vi "OpticsSS.vi"   [LabVIEW 2019]
uses:
  OpticsSS.ctl
types:
  T1 = typedef "OpticsSS.ctl" = enum16{"_Quit_", "Init", "Ready", "HTL", "CCD_shot", "QueueData", "Error Handler", "HTL Error", "CCD Error", "CCDSetup", "Calibration", "BG_Setup", "HTL Paras Setup"}
  T2 = enum16{"CCDSetup", "Calibration", "BGShot", "SequenceShot", "SingleShot", "default"}
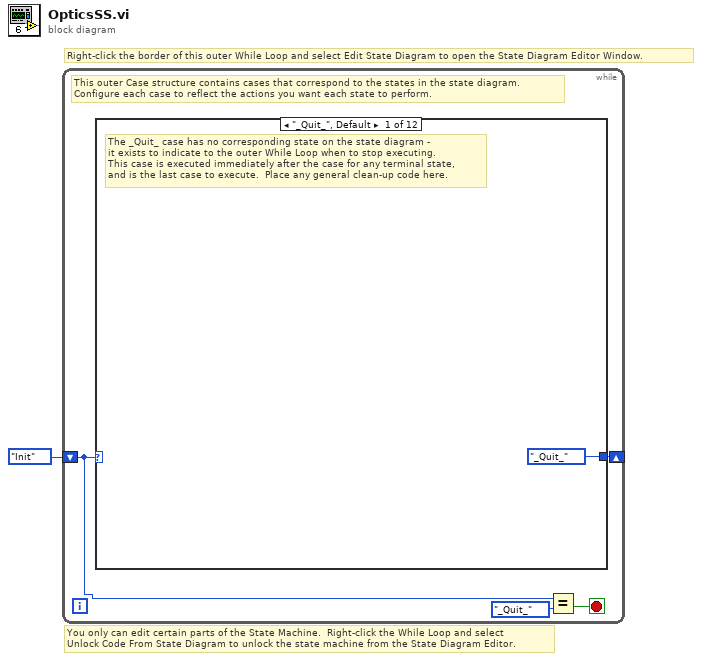
[diagram p0: block diagram]
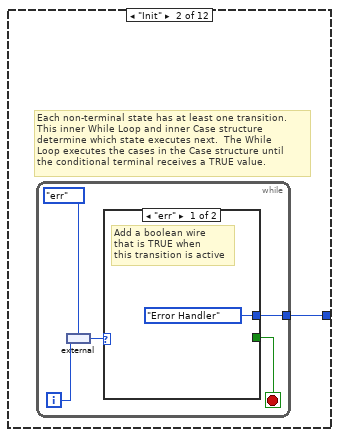
[diagram p2: hidden frame]
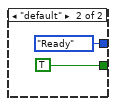
[diagram p3: hidden frame]
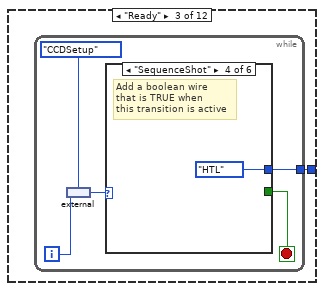
[diagram p4: hidden frame]
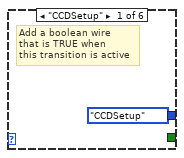
[diagram p5: hidden frame]
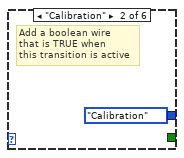
[diagram p6: hidden frame]
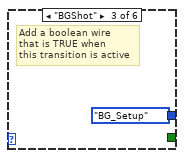
[diagram p7: hidden frame]
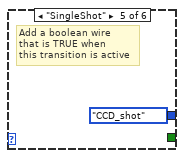
[diagram p8: hidden frame]
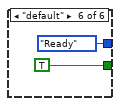
[diagram p9: hidden frame]
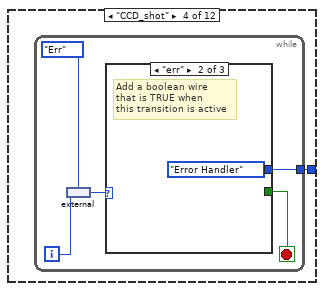
[diagram p10: hidden frame]
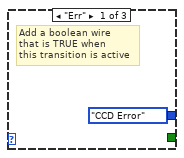
[diagram p11: hidden frame]
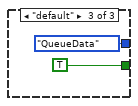
[diagram p12: hidden frame]
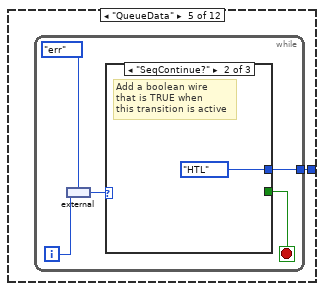
[diagram p13: hidden frame]
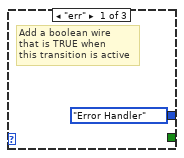
[diagram p14: hidden frame]
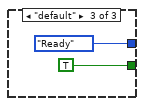
[diagram p15: hidden frame]
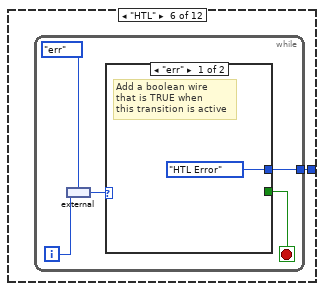
[diagram p16: hidden frame]
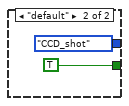
[diagram p17: hidden frame]
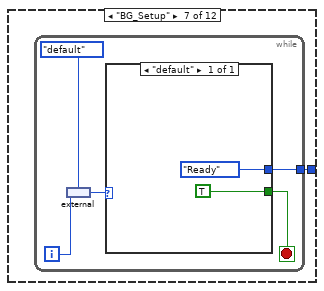
[diagram p18: hidden frame]
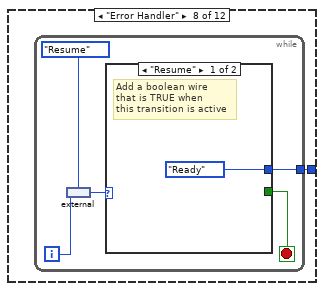
[diagram p19: hidden frame]
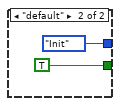
[diagram p20: hidden frame]
diagram:
  # "Right-click the border of this outer While Loop and select Edit State Diagram to open the State Diagram Editor Window."
  # "You only can edit certain parts of the State Machine.  Right-click the While Loop and select \nUnlock Code From State Diagram to unlock the state machine from the State Diagram Editor."
  n1 = while {
    shift-right: [w4] -> _
    shift-left: OpticsSS."Init" -> [w5]
    stop <- w3 stop-if-true
    # "This outer Case structure contains cases that correspond to the states in the state diagram.  \nConfigure each case to reflect the actions you want each state to perform."
    n2 = case shown="\"_Quit_\", Default" w5 {
      tunnel: [OpticsSS."_Quit_" w7 w21 w39 w54 w69 w83 w96 w110 w124 w138 w151] -> w4
      frame "_Quit_", Default {
        # "The _Quit_ case has no corresponding state on the state diagram -\nit exists to indicate to the outer While Loop when to stop executing.\nThis case is executed immediately after the case for any terminal state, \nand is the last case to execute.  Place any general clean-up code here."
      }
      frame "Init" {
        # "Each non-terminal state has at least one transition.\nThis inner While Loop and inner Case structure \ndetermine which state executes next.  The While \nLoop executes the cases in the Case structure until \nthe conditional terminal receives a TRUE value."
        n3 = while {
          tunnel: [w9] -> w7
          i -> [w12]
          stop <- w8 stop-if-true
          n4 = external(enum16{"err", "default"}."err", w12) -> (w10:enum16{"err", "default"})
          n5 = case shown="\"err\"" w10 {
            tunnel: [OpticsSS."Error Handler" OpticsSS."Ready"] -> w9
            tunnel: [_ TRUE] -> w8
            frame "err" {
              # "Add a boolean wire\nthat is TRUE when\nthis transition is active"
            }
            frame "default" {
            }
          }
        }
      }
      frame "Ready" {
        n6 = while {
          tunnel: [w23] -> w21
          i -> [w26]
          stop <- w22 stop-if-true
          n7 = external(T2."CCDSetup", w26) -> (w24:T2)
          n8 = case shown="\"SequenceShot\"" w24 {
            tunnel: [OpticsSS."CCDSetup" OpticsSS."Calibration" OpticsSS."BG_Setup" OpticsSS."HTL" OpticsSS."CCD_shot" OpticsSS."Ready"] -> w23
            tunnel: [_ _ _ _ _ TRUE] -> w22
            frame "CCDSetup" {
              # "Add a boolean wire\nthat is TRUE when\nthis transition is active"
            }
            frame "Calibration" {
              # "Add a boolean wire\nthat is TRUE when\nthis transition is active"
            }
            frame "BGShot" {
              # "Add a boolean wire\nthat is TRUE when\nthis transition is active"
            }
            frame "SequenceShot" {
              # "Add a boolean wire\nthat is TRUE when\nthis transition is active"
            }
            frame "SingleShot" {
              # "Add a boolean wire\nthat is TRUE when\nthis transition is active"
            }
            frame "default" {
            }
          }
        }
      }
      frame "CCD_shot" {
        n9 = while {
          tunnel: [w41] -> w39
          i -> [w44]
          stop <- w40 stop-if-true
          n10 = external(enum16{"Err", "err", "default"}."Err", w44) -> (w42:enum16{"Err", "err", "default"})
          n11 = case shown="\"err\"" w42 {
            tunnel: [OpticsSS."CCD Error" OpticsSS."Error Handler" OpticsSS."QueueData"] -> w41
            tunnel: [_ _ TRUE] -> w40
            frame "Err" {
              # "Add a boolean wire\nthat is TRUE when\nthis transition is active"
            }
            frame "err" {
              # "Add a boolean wire\nthat is TRUE when\nthis transition is active"
            }
            frame "default" {
            }
          }
        }
      }
      frame "QueueData" {
        n12 = while {
          tunnel: [w56] -> w54
          i -> [w59]
          stop <- w55 stop-if-true
          n13 = external(enum16{"err", "SeqContinue?", "default"}."err", w59) -> (w57:enum16{"err", "SeqContinue?", "default"})
          n14 = case shown="\"SeqContinue?\"" w57 {
            tunnel: [OpticsSS."Error Handler" OpticsSS."HTL" OpticsSS."Ready"] -> w56
            tunnel: [_ _ TRUE] -> w55
            frame "err" {
              # "Add a boolean wire\nthat is TRUE when\nthis transition is active"
            }
            frame "SeqContinue?" {
              # "Add a boolean wire\nthat is TRUE when\nthis transition is active"
            }
            frame "default" {
            }
          }
        }
      }
      frame "HTL" {
        n15 = while {
          tunnel: [w71] -> w69
          i -> [w74]
          stop <- w70 stop-if-true
          n16 = external(enum16{"err", "default"}."err", w74) -> (w72:enum16{"err", "default"})
          n17 = case shown="\"err\"" w72 {
            tunnel: [OpticsSS."HTL Error" OpticsSS."CCD_shot"] -> w71
            tunnel: [_ TRUE] -> w70
            frame "err" {
              # "Add a boolean wire\nthat is TRUE when\nthis transition is active"
            }
            frame "default" {
            }
          }
        }
      }
      frame "BG_Setup" {
        n18 = while {
          tunnel: [w85] -> w83
          i -> [w88]
          stop <- w84 stop-if-true
          n19 = external(enum16{"default"}."default", w88) -> (w86:enum16{"default"})
          n20 = case shown="\"default\"" w86 {
            tunnel: [OpticsSS."Ready"] -> w85
            tunnel: [TRUE] -> w84
            frame "default" {
            }
          }
        }
      }
      frame "Error Handler" {
        n21 = while {
          tunnel: [w98] -> w96
          i -> [w101]
          stop <- w97 stop-if-true
          n22 = external(enum16{"Resume", "default"}."Resume", w101) -> (w99:enum16{"Resume", "default"})
          n23 = case shown="\"Resume\"" w99 {
            tunnel: [OpticsSS."Ready" OpticsSS."Init"] -> w98
            tunnel: [_ TRUE] -> w97
            frame "Resume" {
              # "Add a boolean wire\nthat is TRUE when\nthis transition is active"
            }
            frame "default" {
            }
          }
        }
      }
      frame "HTL Error" {
        n24 = while {
          tunnel: [w112] -> w110
          i -> [w115]
          stop <- w111 stop-if-true
          n25 = external(enum16{"Resume", "default"}."Resume", w115) -> (w113:enum16{"Resume", "default"})
          n26 = case shown="\"Resume\"" w113 {
            tunnel: [OpticsSS."HTL" OpticsSS."Error Handler"] -> w112
            tunnel: [_ TRUE] -> w111
            frame "Resume" {
              # "Add a boolean wire\nthat is TRUE when\nthis transition is active"
            }
            frame "default" {
            }
          }
        }
      }
      frame "CCD Error" {
        n27 = while {
          tunnel: [w126] -> w124
          i -> [w129]
          stop <- w125 stop-if-true
          n28 = external(enum16{"Resume", "default"}."Resume", w129) -> (w127:enum16{"Resume", "default"})
          n29 = case shown="\"Resume\"" w127 {
            tunnel: [OpticsSS."CCD_shot" OpticsSS."Error Handler"] -> w126
            tunnel: [_ TRUE] -> w125
            frame "Resume" {
              # "Add a boolean wire\nthat is TRUE when\nthis transition is active"
            }
            frame "default" {
            }
          }
        }
      }
      frame "Calibration" {
        n30 = while {
          tunnel: [w140] -> w138
          i -> [w143]
          stop <- w139 stop-if-true
          n31 = external(enum16{"default"}."default", w143) -> (w141:enum16{"default"})
          n32 = case shown="\"default\"" w141 {
            tunnel: [OpticsSS."Ready"] -> w140
            tunnel: [TRUE] -> w139
            frame "default" {
            }
          }
        }
      }
      frame "CCDSetup" {
        n33 = while {
          tunnel: [w153] -> w151
          i -> [w156]
          stop <- w152 stop-if-true
          n34 = external(enum16{"default"}."default", w156) -> (w154:enum16{"default"})
          n35 = case shown="\"default\"" w154 {
            tunnel: [OpticsSS."Ready"] -> w153
            tunnel: [TRUE] -> w152
            frame "default" {
            }
          }
        }
      }
    }
    n36 = Equal?(x=w5, y=OpticsSS."_Quit_") -> (x = y?=w3:bool)
  }
